vi "Option Parser.vi"(0 "Yokogawa WT1600 in":refnum<class "Yokogawa WT1600.lvclass">, 1 "ID":string, 2 "THD?":bool, 3 "Number of Cards":dbl, 4 "ID cluster.Model":string, 5 "error in (no error)":errorcluster, 7 "Option":string) -> (14 "Yokogawa WT1600 out":refnum<class "Yokogawa WT1600.lvclass">, 19 "error out":errorcluster)   [LabVIEW 2013, in "Universal Power Meter.lvlib" / "Yokogawa WT1600.lvlib" / "Yokogawa WT1600.lvclass"]
uses:
  Yokogawa WT1600.lvclass
  Universal Power Meter class/Universal Power Meter.lvclass
  <vilib>/regexp/Match Regular Expression.xnode
panel:
  out "Array":string[](array[string])
  out "All cards config":string
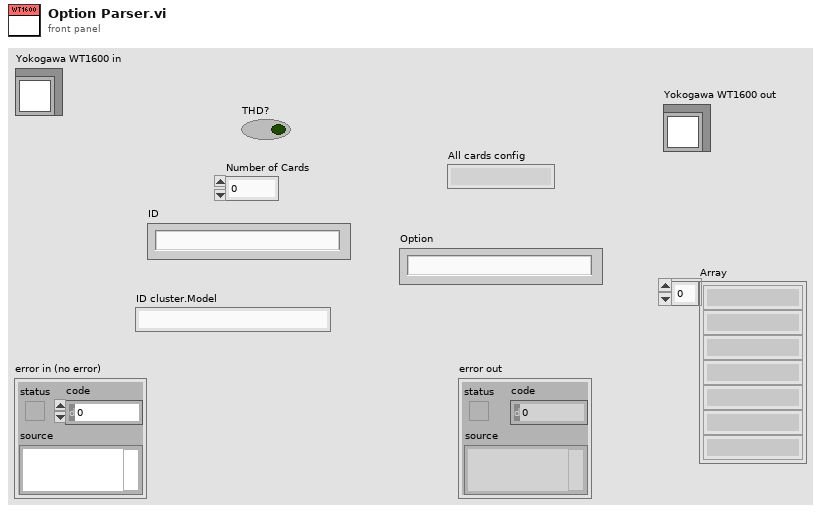
[diagram p1: front panel]
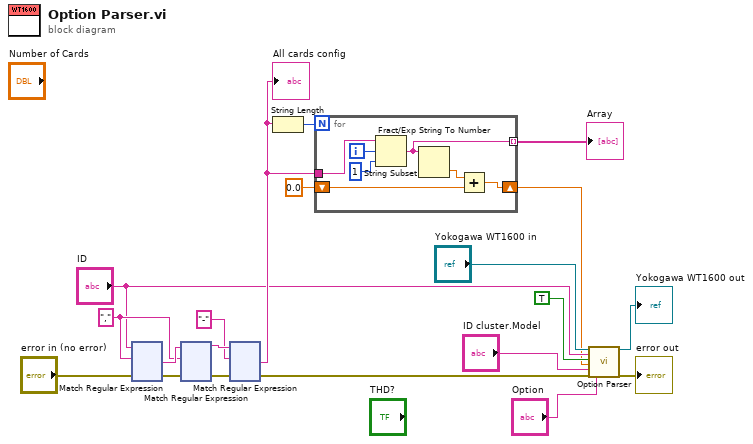
[diagram p0: block diagram]
diagram:
  w14 = "," ("regular expression")
  n1 = xnode "Match Regular Expression"("input string"="ID", "regular expression"=w14, "error in"="error in (no error)") -> ("after match"=w15:string, "error out"=w13:errorcluster)  [unwired: 3 in, 3 out]
  n2 = xnode "Match Regular Expression"("input string"=w15, "regular expression"=w14, "error in"=w13) -> ("before match"=w12:string, "error out"=w10:errorcluster)  [unwired: 3 in, 3 out]
  n3 = xnode "Match Regular Expression"("input string"=w12, "regular expression"="-", "error in"=w10) -> ("after match"=w8:string, "error out"=w1:errorcluster)  [unwired: 3 in, 3 out]
  "All cards config" <- w8
  n4 = String Length(string=w8) -> (length=w9:i32)
  n5 = for {
    N: w9 -> [_]
    tunnel: w8 -> [w27]
    tunnel: [w24] -> w7 mode=indexing
    shift-right: [w21] -> w4
    shift-left: 0.0 -> [w22]
    i -> [w26]
    n6 = String Subset(string=w27, offset (0)=w26, length (rest)=1 ("length (rest)")) -> (substring=w24:string)
    n7 = Fract/Exp String To Number(string=w24) -> (number=w23:dbl)  [unwired: 3 in, 1 out]
    n8 = Add(x=w23, y=w22) -> (x+y=w21:dbl)
  }
  "Array" <- w7
  n9 = call-parent "Option Parser.vi"("Universal Power Meter in"="Yokogawa WT1600 in", "ID"="ID", "THD?"=TRUE, "Number of Cards"=w4, "ID cluster.Model"="ID cluster.Model", "error in (no error)"=w1, "Option"="Option") -> ("Universal Power Meter out"=→"Yokogawa WT1600 out":refnum<class "Yokogawa WT1600.lvclass">, "error out"=→"error out":errorcluster)  [unwired: 11 in]
